vi "Set Values.vi"(8 "error in (no error)":errorcluster, 9 "Settle Time":dbl, 10 "Step Temp":dbl, 11 "Target Step in":refnum<class "Target Step.lvclass">) -> (0 "error out":errorcluster, 3 "Target Step out":refnum<class "Target Step.lvclass">)   [LabVIEW 2018, in "Temp Recipe.lvlib" / "Target Step.lvclass"]
uses:
  Target Step.lvclass
  C:/dev/source/Systems/NI Week/Temperature Recipe/Temp Recipe/Recipe Step/Recipe Step.lvclass
  Target Step.lvclass/Target Step.ctl
  Recipe Step/Recipe Step.lvclass
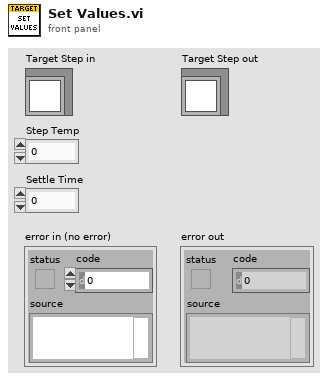
[diagram p1: front panel]
types:
  T1 = typedef "Temp Recipe.lvlib/Target Step.lvclass/Ref Data.ctl" = cluster{"Step Temp":dbl, "Settle Time":dbl}
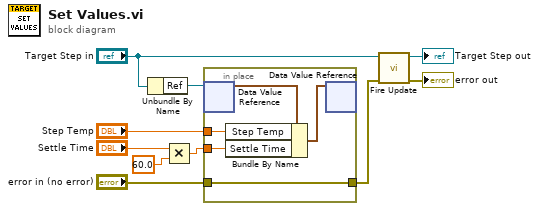
[diagram p0: block diagram]
diagram:
  n1 = Unbundle By Name("Target Step in") -> ("Ref"=w10:refnum<data-value>)
  n2 = Multiply(x="Settle Time", y=60.0) -> (x*y=w1:dbl)
  n3 = in-place {
    in-place-border: "Step Temp" -> [w13]
    in-place-border: w1 -> [w12]
    in-place-border: "error in (no error)" -> [w11]
    in-place-border: [w11] -> w9
    n4 = in-place-dvr #1(w10) -> (w15:T1)  [unwired: 1 out]
    n5 = Bundle By Name(cluster=w15, "Step Temp"=w13, "Settle Time"=w12) -> (w14:T1)
    n6 = in-place-dvr #1(w14) -> ()  [unwired: 2 out]
  }
  n7 = call "Fire Update.vi"("error in (no error)"=w9, "Recipe Step in"="Target Step in") -> ("error out"=→"error out":errorcluster, "Recipe Step out"=→"Target Step out":refnum<class "Target Step.lvclass">)  [unwired: 8 in]
